vi "Output Graph Data.vi"(10 "Experiment State":T1={"Send Trigger 3"=FALSE, "error"={"status"=FALSE, "code"=0, "source"=""}, "Digitizer DAQmx Tasks"={"TaskArray"=[]}, "Digitizer Settings"={"6133 Digitizer Channels"=[], "Global Edge Type"=10280, "Total Samples"=[], "Pre-Trigger Samples"=[], "Sample Rate"=[], "Trigger Sources"=[], "Voltage Ranges"=[], "Channel Names"=[], "Active"=[], "Samples to remove"=[], "Start Time"=[], "End Time"=[]}, "Timing Card 2 Fast Outputs"=[{"Delay (s)"=2.559999942779541, "Pulse width (s)"=0.009999999776482582, "Active"=TRUE, "Channel Name"="Fiber 8", "counter"="PXI1Slot8/ctr7"}], "Synchronization Card Settings"={"Position"="PXI1Slot2", "source terminal"="GlobalSoftwareTrigger"}, "Digitizer Data"=[], "Next Shot#"="0", "Timing Card 1 Settings"={"Slot 8 Trigger Source"="", "Clock Source"="", "Trigger Channel Tasks"=[]}, "Timing Card 2 Settings"={"Clock Source"="", "Slot 9 Trigger Source"="", "Trigger Channel Tasks"=[]}, "Timing Card 1 Fast Outputs"=[{"Delay (s)"=2.559999942779541, "Pulse width (s)"=0.009999999776482582, "Active"=TRUE, "Channel Name"="Fiber 8", "counter"="PXI1Slot8/ctr7"}], "System Message"="", "User Shot Notes"=""} {"Timing Card 1 Fast Outputs"."Pulse width (s)" format="%.3p"; "Timing Card 1 Fast Outputs"."Delay (s)" format="%.3p"; "Timing Card 2 Fast Outputs"."Pulse width (s)" format="%.3p"; "Timing Card 2 Fast Outputs"."Delay (s)" format="%.3p"; "Digitizer Settings"."Sample Rate" format="%#_3p"; "Digitizer Settings"."Global Edge Type" items=["Rising"=10280, "Falling"=10171]}, 11 "Ctl Refnum":refnum<vi>) -> ()   [LabVIEW 2013]
doc: "Takes Channel Data from each channel and outputs to graphs on front panel"
uses:
  Controls/ExperimentStateCluster.ctl
panel:
  out "XY Graph":cluster{dbl[], "Y":dbl[]}(graph)
  # "Channel Settings"
  # "Card Wide Settings"
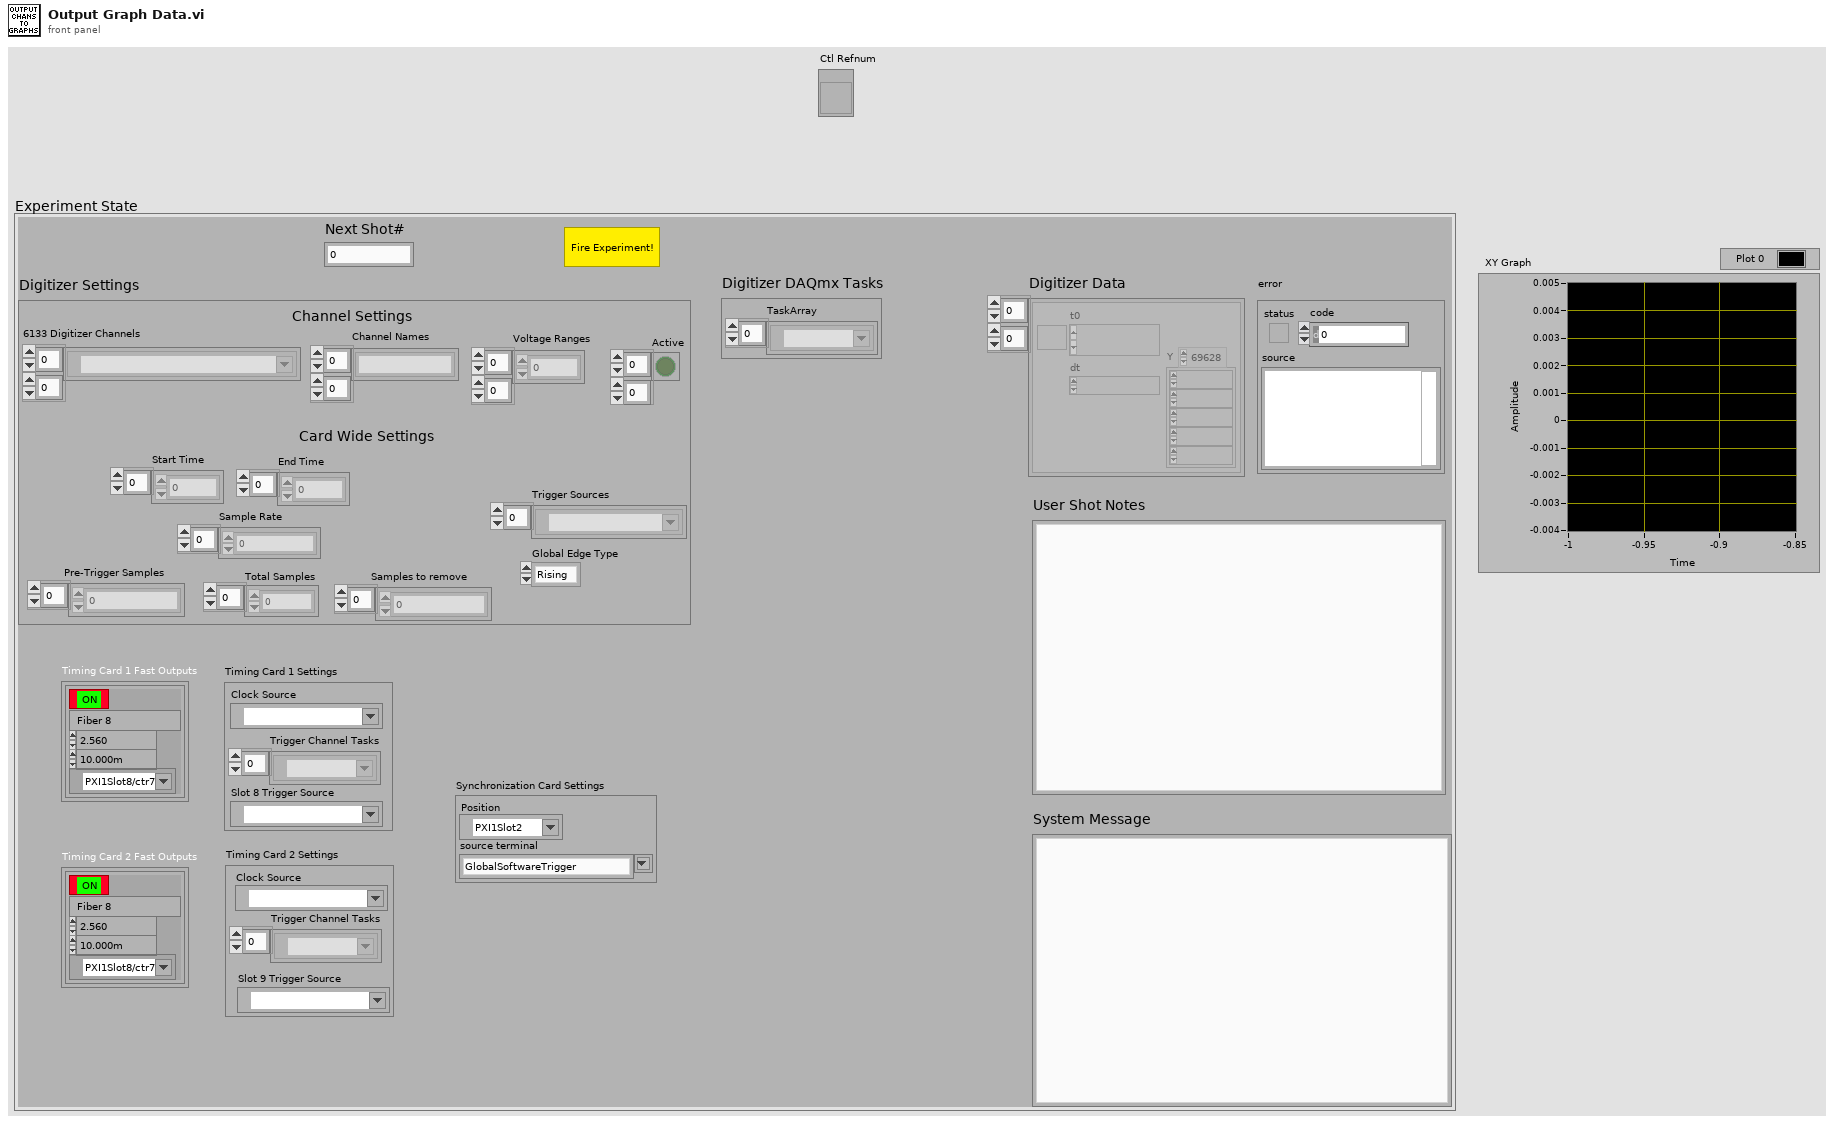
[diagram p1: front panel]
types:
  T1 = typedef "ExperimentStateCluster.ctl" = cluster{"Send Trigger 3":bool, "error":errorcluster, "Digitizer DAQmx Tasks":cluster{"TaskArray":refnum<k21>[]}, "Digitizer Settings":cluster{"6133 Digitizer Channels":tag[][], "Global Edge Type":i32, "Total Samples":i32[], "Pre-Trigger Samples":u32[], "Sample Rate":dbl[], "Trigger Sources":tag[], "Voltage Ranges":dbl[][], "Channel Names":string[][], "Active":bool[][], "Samples to remove":u32[], "Start Time":dbl[], "End Time":dbl[]}, "Timing Card 2 Fast Outputs":cluster{"Delay (s)":dbl, "Pulse width (s)":dbl, "Active":bool, "Channel Name":string, "counter":tag}[], "Synchronization Card Settings":cluster{"Position":refnum<k15>, "source terminal":string}, "Digitizer Data":waveform(dbl)[][], "Next Shot#":string, "Timing Card 1 Settings":cluster{"Slot 8 Trigger Source":tag, "Clock Source":tag, "Trigger Channel Tasks":refnum<k21>[]}, "Timing Card 2 Settings":cluster{"Clock Source":tag, "Slot 9 Trigger Source":tag, "Trigger Channel Tasks":refnum<k21>[]}, "Timing Card 1 Fast Outputs":cluster{"Delay (s)":dbl, "Pulse width (s)":dbl, "Active":bool, "Channel Name":string, "counter":tag}[], "System Message":string, "User Shot Notes":string}
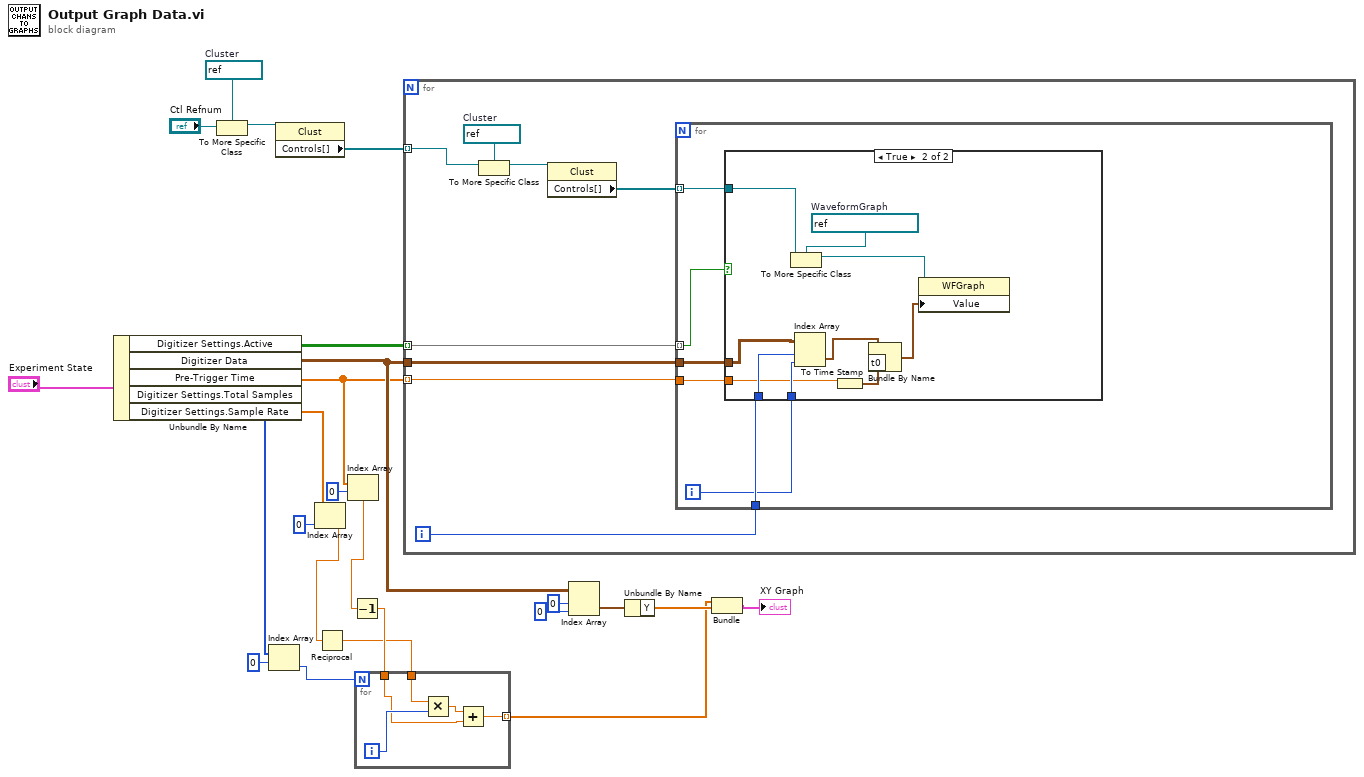
[diagram p0: block diagram]
diagram:
  w23 = refnum<vi> refnum  # Cluster
  n1 = Unbundle By Name("Experiment State") -> ("Digitizer Settings.Active"=w19:bool[][], "Digitizer Data"=w18:waveform(dbl)[][], "Pre-Trigger Time"=w9:dbl[], "Digitizer Settings.Total Samples"=w6:i32[], "Digitizer Settings.Sample Rate"=w12:dbl[])
  n2 = To More Specific Class(target class=w23, reference="Ctl Refnum") -> (specific class reference=w22:refnum<vi>)  [unwired: 1 in, 1 out]
  n3 = Index Array(array=w6, index=0) -> (element=w4:i32)
  n4 = property class="Clust"(reference=w22) -> ("Controls[]"=w21:refnum<vi>[])  [unwired: 1 in, 2 out]
  n5 = Index Array(array=w12, index=0) -> (element=w10:dbl)
  n6 = Reciprocal(x=w10) -> (1/x=w2:dbl)
  n7 = Index Array(array=w9, index=0) -> (element=w7:dbl)
  n8 = Decrement(x=w7) -> (x-1=w3:dbl)
  n9 = for {
    N: w4 -> [_]
    tunnel: w3 -> [w26]
    tunnel: w2 -> [w29]
    tunnel: [w25] -> w1 mode=indexing
    i -> [w28]
    n10 = Multiply(x=w29, y=w28) -> (x*y=w27:dbl)
    n11 = Add(x=w27, y=w26) -> (x+y=w25:dbl)
  }
  n12 = for {
    tunnel: w21 -> [w37] mode=indexing
    tunnel: w18 -> [w33]
    tunnel: w19 -> [w32] mode=indexing
    tunnel: w9 -> [w30] mode=indexing
    i -> [w31]
    w36 = refnum<vi> refnum  # Cluster
    n13 = To More Specific Class(target class=w36, reference=w37) -> (specific class reference=w35:refnum<vi>)  [unwired: 1 in, 1 out]
    n14 = property class="Clust"(reference=w35) -> ("Controls[]"=w34:refnum<vi>[])  [unwired: 1 in, 2 out]
    n15 = for {
      tunnel: w34 -> [w43] mode=indexing
      tunnel: w33 -> [w42]
      tunnel: w32 -> [w41] mode=indexing
      tunnel: w31 -> [w40]
      tunnel: w30 -> [w38]
      i -> [w39]
      n16 = case shown="True" w41 {
        tunnel: w43 -> [_ w53]
        tunnel: w42 -> [_ w50]
        tunnel: w40 -> [_ w49]
        tunnel: w39 -> [_ w48]
        tunnel: w38 -> [_ w45]
        frame False {
        }
        frame True {
          w52 = refnum<vi> refnum  # WaveformGraph
          n17 = To More Specific Class(target class=w52, reference=w53) -> (specific class reference=w51:refnum<vi>)  [unwired: 1 in, 1 out]
          n18 = Index Array(array=w50, index (row)=w49, index (col)=w48) -> (element=w46:waveform(dbl))
          n19 = To Time Stamp(1:w45) -> (0:w44:timestamp)
          n20 = Bundle By Name(cluster=w46, "t0"=w44) -> (w47:waveform(dbl))
          n21 = property class="WFGraph"(reference=w51, "Value"=w47) -> ()  [unwired: 1 in, 2 out]
        }
      }
    }
  }
  n22 = Index Array(array=w18, index (row)=0, index (col)=0 ("disabled index (col)")) -> (element=w15:waveform(dbl))
  n23 = Unbundle By Name(w15) -> ("Y"=w13:dbl[])
  n24 = Bundle(w1, "Y"=w13) -> (→"XY Graph":cluster{dbl[], "Y":dbl[]})  [unwired: 1 in]
